vi "createRangeString.vi"(6 "range (0.000)":dbl, 8 "error in (no error)":errorcluster, 9 "Function":string, 10 "Channel (Channel A)":T1, 11 "K2602 in":refnum<class "K2602.lvclass">) -> (0 "error out":errorcluster, 2 "Limit string":string, 3 "K2602 out":refnum<class "K2602.lvclass">)   [LabVIEW 2009, in "Hardware.lvlib" / "Channels.lvlib" / "K2602.lvclass"]
uses:
  K2602.lvclass
  <instrlib>/Keithley 2600 Series/Public/Channel.ctl
  K2602.lvclass/K2602.ctl
  <instrlib>/Keithley 2600 Series/Keithley 2600 Series.lvlib
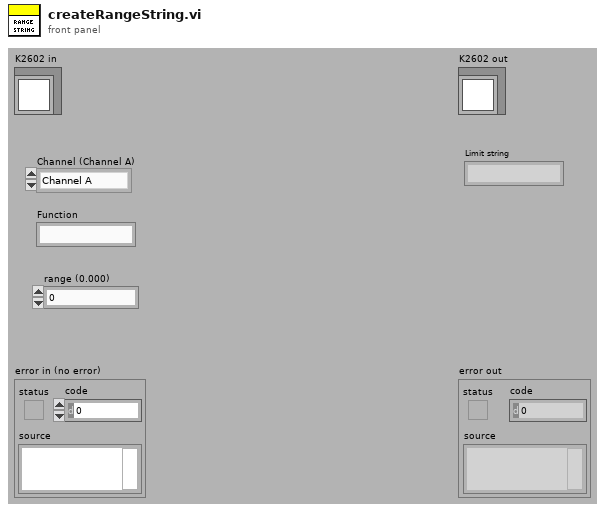
[diagram p1: front panel]
types:
  T1 = typedef "Keithley 2600 Series.lvlib/Channel.ctl" = enum32{"Channel A", "Channel B"}
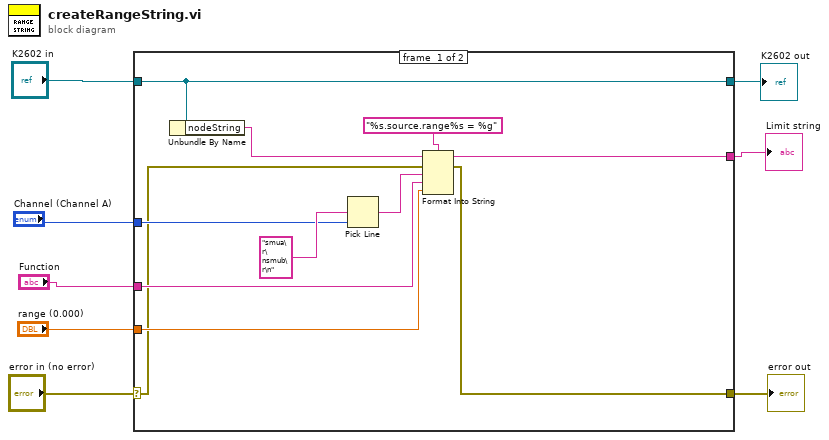
[diagram p0: block diagram]
diagram:
  n1 = case shown="No Error" "error in (no error)" {
    selector: "error in (no error)" -> [w10 w21]
    tunnel: [w9 w21] -> w7
    tunnel: [w13 w20] -> w5
    tunnel: "K2602 in" -> [w13 w20]
    tunnel: "range (0.000)" -> [w15 _]
    tunnel: "Function" -> [w14 _]
    tunnel: "Channel (Channel A)" -> [w16 _]
    tunnel: [w11 _] -> w1
    frame #0 {
      n2 = Unbundle By Name(w13) -> ("nodeString"=w12:string)
      n3 = Pick Line(multi-line string="smua\r\nsmub\r\n" ("options"), line index=w16) -> (output string=w17:string)  [unwired: 1 out]
      n4 = Format Into String(format string="%s.source.range%s = %g", initial string=w12, error in=w10, w17, w14, w15) -> (resulting string=w11:string, error out=w9:errorcluster)
    }
    frame #1 {
    }
  }
  "error out" <- w7
  "K2602 out" <- w5
  "Limit string" <- w1
